vi "Setup Power Supplies.vi"(10 "DC Supplies":refnum<class "Instrument.lvclass">[](array[class]), 11 "AC Supplies":refnum<class "Instrument.lvclass">[](array[class])) -> (0 "error out":errorcluster)   [LabVIEW 2015, in "Instrument Close.lvclass"]
uses:
  Instrument Close.lvclass
  Classes/Instruments/Instrument/Class/Instrument.lvclass
  Classes/Instruments/Power Supply/Class/Power Supply.lvclass
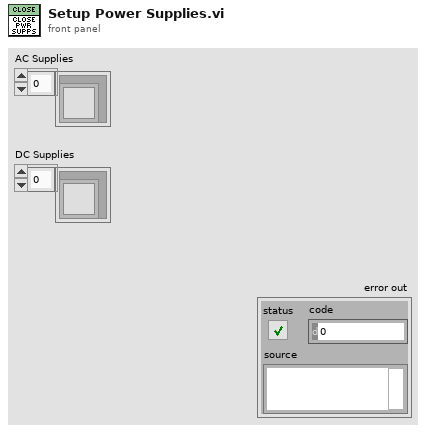
[diagram p1: front panel]
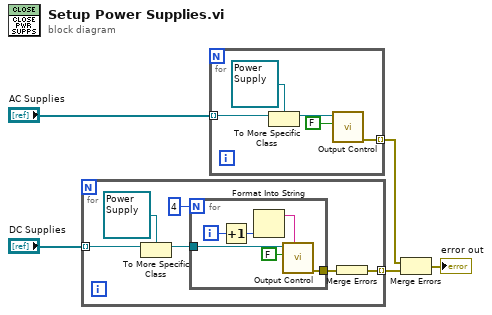
[diagram p0: block diagram]
diagram:
  n1 = for {
    tunnel: "DC Supplies" -> [w9] mode=indexing
    tunnel: [w7] -> w3 mode=indexing
    n2 = To More Specific Class(target class=refnum<class "Power Supply.lvclass"> refnum ("Acrobat Template in"), reference=w9) -> (specific class reference=w10:refnum<class "Power Supply.lvclass">)  [unwired: 1 in, 1 out]
    n3 = for {
      N: 4 -> [_]
      tunnel: w10 -> [w17]
      tunnel: [w15] -> w8
      i -> [w14]
      n4 = Increment(x=w14) -> (x+1=w12:i32)
      n5 = Format Into String(w12) -> (resulting string=w13:string)  [unwired: 3 in, 1 out]
      n6 = call-dynamic "Output Control.vi"("Channel (\"1\")"=w13, "Enabled"=FALSE, "Acrobat Template in"=w17) -> ("error out"=w15:errorcluster)  [unwired: 7 in, 1 out]
    }
    n7 = Merge Errors(w8) -> (w7:errorcluster)
  }
  n8 = for {
    tunnel: "AC Supplies" -> [w19] mode=indexing
    tunnel: [w18] -> w2 mode=indexing
    n9 = To More Specific Class(target class=refnum<class "Power Supply.lvclass"> refnum ("Acrobat Template in"), reference=w19) -> (specific class reference=w21:refnum<class "Power Supply.lvclass">)  [unwired: 1 in, 1 out]
    n10 = call-dynamic "Output Control.vi"("Enabled"=FALSE, "Acrobat Template in"=w21) -> ("error out"=w18:errorcluster)  [unwired: 8 in, 1 out]
  }
  n11 = Merge Errors(w2, w3) -> (→"error out":errorcluster)
